vi "COM test.vi"() -> ()   [LabVIEW 2023]
panel:
  in  "Message Based Settings:Termination Character":u8=13 format="%x"
  out "return count":u32
  out "read buffer":string
  out "VISA resource name out":refnum<visa-resource-name>
  out "error out":errorcluster
  in  "byte count":u32=256
  in  "error in (no error)":errorcluster
  in  "write buffer":string="*IDN?\n"
  in  "VISA resource name":refnum<visa-resource-name>
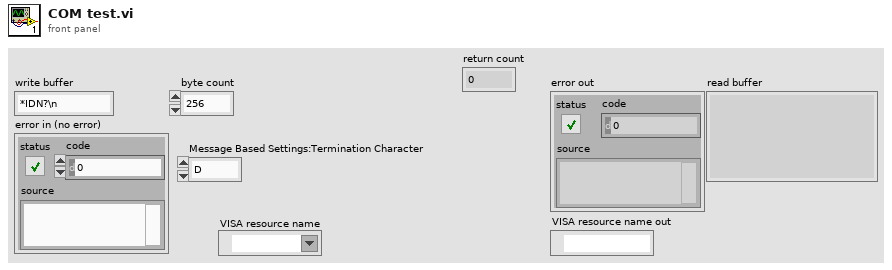
[diagram p1: front panel]
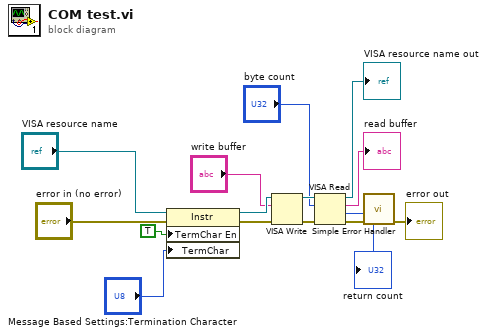
[diagram p0: block diagram]
diagram:
  n1 = property class="Instr"(reference="VISA resource name", error in="error in (no error)", "TermChar En"=TRUE ("Message Based Settings:Termination Character Enable"), "TermChar"="Message Based Settings:Termination Character") -> (reference out=w14:refnum<visa-resource-name>, error out=w11:errorcluster)
  n2 = VISA Write(VISA resource name=w14, write buffer="write buffer", error in (no error)=w11) -> (VISA resource name out=w7:refnum<visa-resource-name>, error out=w8:errorcluster)  [unwired: 1 out]
  n3 = VISA Read(VISA resource name=w7, byte count="byte count", error in (no error)=w8) -> (VISA resource name out=→"VISA resource name out":refnum<visa-resource-name>, read buffer=→"read buffer":string, return count=→"return count":u32, error out=w5:errorcluster)
  n4 = call <vilib>:"Simple Error Handler.vi"("error in (no error)"=w5) -> ("error out"=→"error out":errorcluster)  [unwired: 4 in, 4 out]
